vi "Measure Single Digital.vi"(8 "error in":errorcluster, 10 "task/channels in":refnum<k21>) -> (0 "error out":errorcluster, 1 "data":bool, 2 "task out":refnum<k21>)   [LabVIEW 2021]
uses:
  <vilib>/DAQmx/read.llb/DAQmx Read (Digital Bool 1Line 1Point).vi
  <vilib>/DAQmx/miscellaneous.llb/DAQmx Fill In Error Info.vi
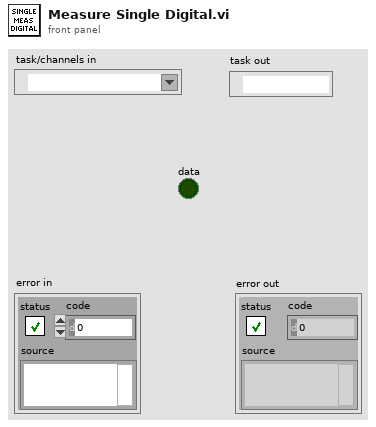
[diagram p1: front panel]
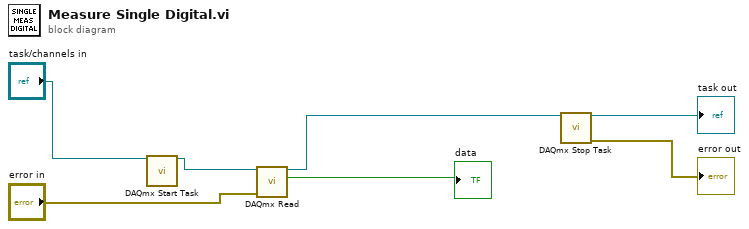
[diagram p0: block diagram]
diagram:
  n1 = call <vilib>:"DAQmx Start Task.vi"("task/channels in"="task/channels in") -> ("task out"=w6:refnum<k21>)  [unwired: 13 in, 1 out]
  n2 = call-poly <vilib>:"DAQmx Read.vi"("task/channels in"=w6, "error in"="error in") -> ("task out"=w4:refnum<k21>, "data"=→"data":bool)  [unwired: 11 in, 1 out]
  n3 = call <vilib>:"DAQmx Stop Task.vi"("task/channels in"=w4) -> ("task out"=→"task out":refnum<k21>, "error out"=→"error out":errorcluster)  [unwired: 13 in]
